vi "Test Speaker Traverse Logic.vi"() -> ()   [LabVIEW 2018]
panel:
  in  "x":i32
  out "Waveform Chart":i32(graph)
  out "Numeric Control":i32
  out "i":i32
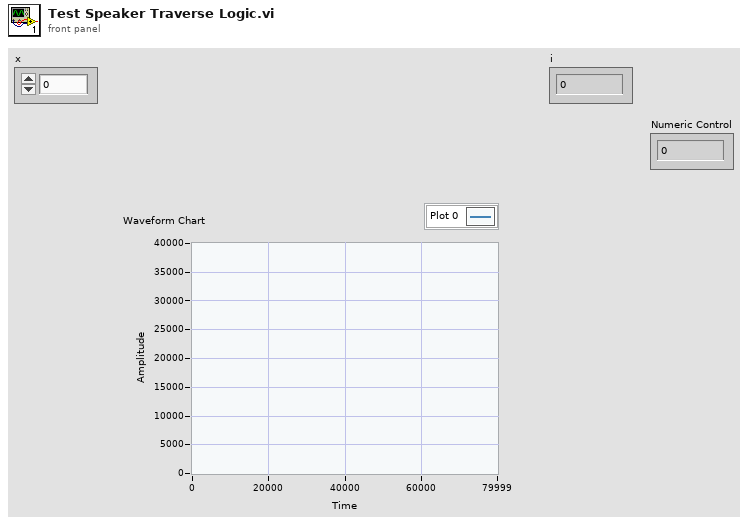
[diagram p1: front panel]
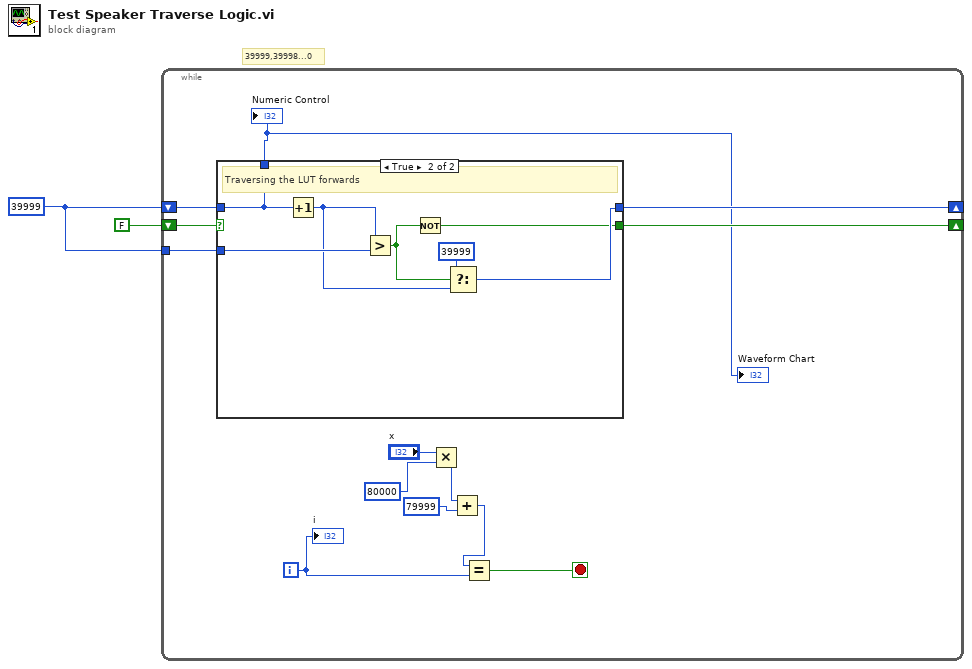
[diagram p0: block diagram]
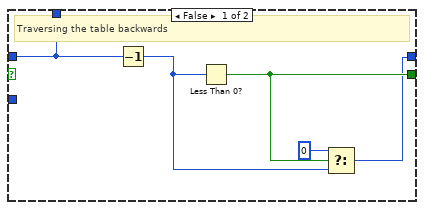
[diagram p2: hidden frame]
diagram:
  w1 = 39999
  # "39999,39998...0"
  n1 = while {
    shift-right: [w13] -> _
    shift-left: FALSE -> [w14]
    shift-right: [w9] -> _
    shift-left: w1 -> [w15]
    tunnel: w1 -> [w10]
    i -> [w12]
    stop <- w11 stop-if-true
    n2 = case "Check where we are in the chirp" shown="True" w14 {
      tunnel: w15 -> [w20 w25]
      tunnel: [w19 w21] -> w13
      tunnel: [w20 w25] -> w8
      tunnel: [w17 w27] -> w9
      tunnel: w10 -> [_ w26]
      frame False {
        # "Traversing the table backwards"
        n3 = Decrement(x=w20) -> (x-1=w18:i32)
        n4 = Less Than 0?(x=w18) -> (x < 0?=w19:bool)
        n5 = Select(t=0, s=w19, f=w18) -> (s? t:f=w17:i32)
      }
      frame True {
        # "Traversing the LUT forwards"
        n6 = Increment(x=w25) -> (x+1=w24:i32)
        n7 = Greater?(x=w24, y=w26) -> (0:w22:bool)
        n8 = Not(x=w22) -> (.not. x?=w21:bool)
        n9 = Select(t=39999, s=w22, f=w24) -> (s? t:f=w27:i32)
      }
    }
    "Numeric Control" <- w8
    "Waveform Chart" <- w8
    n10 = Multiply(x="x", y=80000 ("x")) -> (x*y=w3:i32)
    n11 = Add(x=w3, y=79999 ("x")) -> (x+y=w6:i32)
    n12 = Equal?(x=w6, y=w12) -> (x = y?=w11:bool)
    "i" <- w12
  }
